vi "X stage safety.vi"(7 "new position":dbl format="%#_13g", 8 "Error In":errorcluster, 10 "Table Stages":T1={"X Stage"={"Position"=0.0, "Is.Enabled?"=FALSE, "Is.Connected?"=FALSE, "Device SN"="45876539", "AccelerationMaximum"=0.0, "VelocityMaximum"=0.0, "Acceleration"=0.0, "Velocity"=0.0, "waitTimeout (ms)"=0, "Model"=enum."None", "Is.Homed?"=FALSE, "MOVE"=FALSE}, "Y Stage"={"Position"=0.0, "Is.Enabled?"=FALSE, "Is.Connected?"=FALSE, "Device SN"="45876539", "AccelerationMaximum"=0.0, "VelocityMaximum"=0.0, "Acceleration"=0.0, "Velocity"=0.0, "waitTimeout (ms)"=0, "Model"=enum."None", "Is.Homed?"=FALSE, "MOVE"=FALSE}, "Z Stage"={"Position"=0.0, "Is.Enabled?"=FALSE, "Is.Connected?"=FALSE, "Device SN"="45876539", "AccelerationMaximum"=0.0, "VelocityMaximum"=0.0, "Acceleration"=0.0, "Velocity"=0.0, "waitTimeout (ms)"=0, "Model"=enum."None", "Is.Homed?"=FALSE, "MOVE"=FALSE}, "Attenuator"={"Position"=0.0, "Is.Enabled?"=FALSE, "Is.Connected?"=FALSE, "Device SN"="45876539", "AccelerationMaximum"=0.0, "VelocityMaximum"=0.0, "Acceleration"=0.0, "Velocity"=0.0, "waitTimeout (ms)"=0, "Model"=enum."None", "Is.Homed?"=FALSE, "MOVE"=FALSE}}) -> (0 "Error Out":errorcluster, 1 "crash?":bool, 2 "Table Stages [out]":T1={"X Stage"={"Position"=0.0, "Is.Enabled?"=FALSE, "Is.Connected?"=FALSE, "Device SN"="45876539", "AccelerationMaximum"=0.0, "VelocityMaximum"=0.0, "Acceleration"=0.0, "Velocity"=0.0, "waitTimeout (ms)"=0, "Model"=enum."None", "Is.Homed?"=FALSE, "MOVE"=FALSE}, "Y Stage"={"Position"=0.0, "Is.Enabled?"=FALSE, "Is.Connected?"=FALSE, "Device SN"="45876539", "AccelerationMaximum"=0.0, "VelocityMaximum"=0.0, "Acceleration"=0.0, "Velocity"=0.0, "waitTimeout (ms)"=0, "Model"=enum."None", "Is.Homed?"=FALSE, "MOVE"=FALSE}, "Z Stage"={"Position"=0.0, "Is.Enabled?"=FALSE, "Is.Connected?"=FALSE, "Device SN"="45876539", "AccelerationMaximum"=0.0, "VelocityMaximum"=0.0, "Acceleration"=0.0, "Velocity"=0.0, "waitTimeout (ms)"=0, "Model"=enum."None", "Is.Homed?"=FALSE, "MOVE"=FALSE}, "Attenuator"={"Position"=0.0, "Is.Enabled?"=FALSE, "Is.Connected?"=FALSE, "Device SN"="45876539", "AccelerationMaximum"=0.0, "VelocityMaximum"=0.0, "Acceleration"=0.0, "Velocity"=0.0, "waitTimeout (ms)"=0, "Model"=enum."None", "Is.Homed?"=FALSE, "MOVE"=FALSE}})   [LabVIEW 2018]
uses:
  Controls/Translation Stage Parameters.ctl
  Hardware Mfg/Thorlabs Translation Stages/Controls/Translation Stage Cluster.ctl
  Controls/Translation Stage Types.ctl
  Controls/Set Get Controls.ctl
  Hardware Mfg/Thorlabs Translation Stages/Controls/Motion Translation Module Control2.ctl
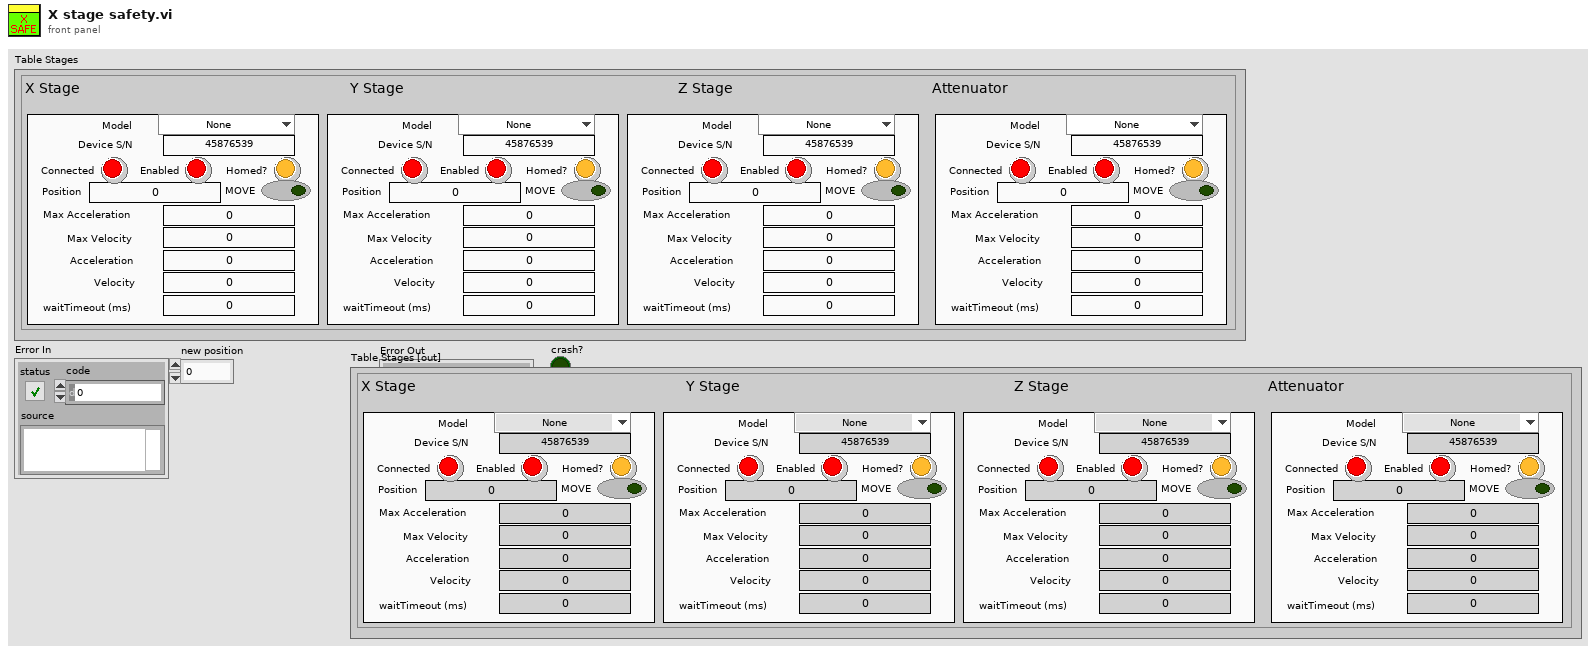
[diagram p1: front panel]
types:
  T1 = typedef "Translation Stage Parameters.ctl" = cluster{"X Stage":T2, "Y Stage":T2, "Z Stage":T2, "Attenuator":T2}
  T2 = typedef "Translation Stage Cluster.ctl" = cluster{"Position":dbl, "Is.Enabled?":bool, "Is.Connected?":bool, "Device SN":string, "AccelerationMaximum":dbl, "VelocityMaximum":dbl, "Acceleration":dbl, "Velocity":dbl, "waitTimeout (ms)":i32, "Model":T3, "Is.Homed?":bool, "MOVE":bool}
  T3 = typedef "Translation Stage Types.ctl" = enum16{"None", "Thorlabs LTS", "Thorlabs MLJ"}
  T4 = typedef "Motion Translation Module Control2.ctl" = enum16{"Init", "Home", "Status", "Velocity/Accel", "Position", "Jog", "Stop", "Uninit", "Enable", "Disable"}
  T5 = typedef "Set Get Controls.ctl" = enum16{"Set", "Get"}
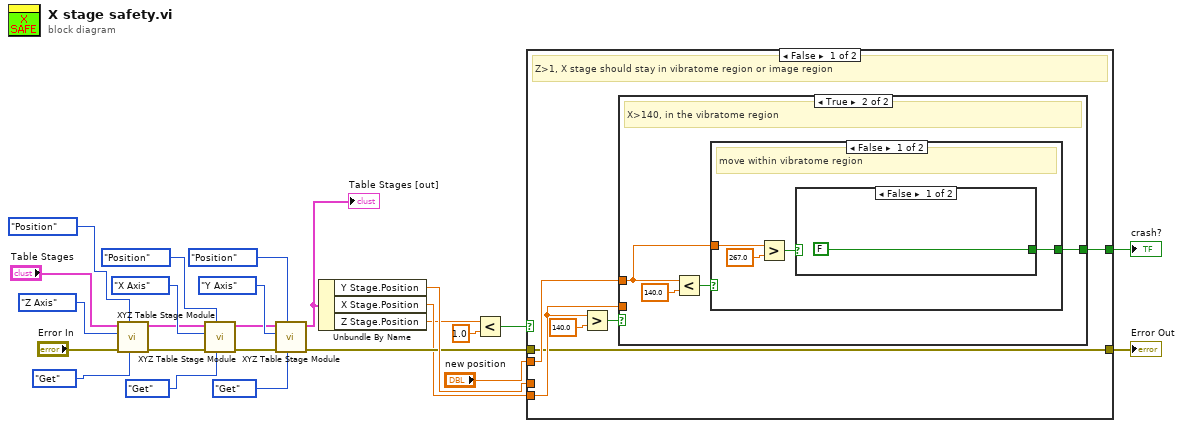
[diagram p0: block diagram]
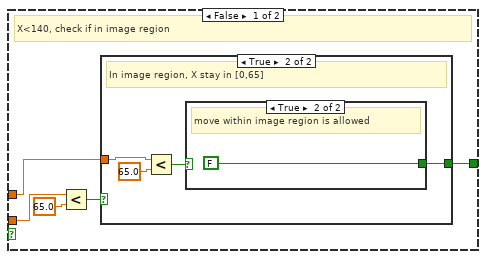
[diagram p2: hidden frame]
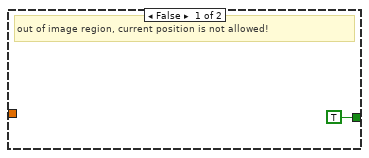
[diagram p3: hidden frame]
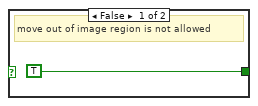
[diagram p4: hidden frame]
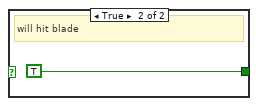
[diagram p5: hidden frame]
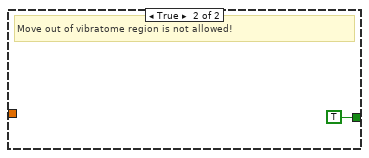
[diagram p6: hidden frame]
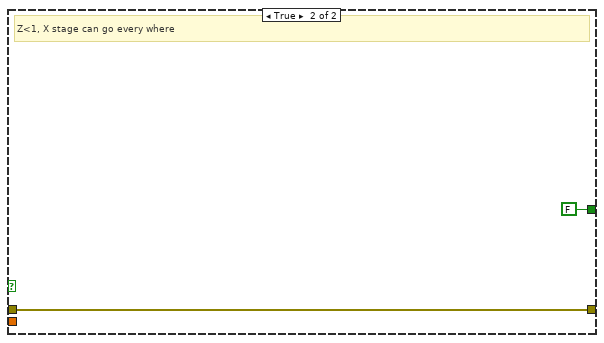
[diagram p7: hidden frame]
diagram:
  n1 = call "XYZ Table Stage Module.vi"("Set/Get"=Set_Get_Controls."Get", "Action"=Motion_Translation_Module_Control2."Position", "Error In"="Error In", "Axis"=enum16{"X Axis", "Y Axis", "Z Axis"}."Z Axis", "Table Stages"="Table Stages") -> ("Error Out"=w18:errorcluster, "Table Stages [out]"=w4:T1)  [unwired: 5 in]
  n2 = call "XYZ Table Stage Module.vi"("Set/Get"=Set_Get_Controls."Get", "Action"=Motion_Translation_Module_Control2."Position", "Error In"=w18, "Axis"=enum16{"X Axis", "Y Axis", "Z Axis"}."X Axis", "Table Stages"=w4) -> ("Error Out"=w14:errorcluster, "Table Stages [out]"=w3:T1)  [unwired: 5 in]
  n3 = call "XYZ Table Stage Module.vi"("Set/Get"=Set_Get_Controls."Get", "Action"=Motion_Translation_Module_Control2."Position", "Error In"=w14, "Axis"=enum16{"X Axis", "Y Axis", "Z Axis"}."Y Axis", "Table Stages"=w3) -> ("Error Out"=w6:errorcluster, "Table Stages [out]"=w13:T1)  [unwired: 5 in]
  "Table Stages [out]" <- w13
  n4 = Unbundle By Name(w13) -> ("Y Stage.Position"=w9:dbl, "X Stage.Position"=w2:dbl, "Z Stage.Position"=w1:dbl)
  n5 = Less?(x=w1, y=1.0) -> (x < y?=w11:bool)
  n6 = case shown="False" w11 {
    tunnel: "new position" -> [w29 _]
    tunnel: w9 -> [_ _]
    tunnel: [w27 FALSE] -> w8
    tunnel: w2 -> [w28 _]
    tunnel: w6 -> [w26 w55]
    tunnel: [w26 w55] -> w5
    frame False {
      # "Z>1, X stage should stay in vibratome region or image region"
      n7 = Greater?(x=w28, y=140.0) -> (0:w30:bool)
      n8 = case shown="True" w30 {
        tunnel: w29 -> [w32 w44]
        tunnel: [w33 w45] -> w27
        tunnel: w28 -> [w36 _]
        frame False {
          # "X<140, check if in image region"
          n9 = Less?(x=w36, y=65.0) -> (x < y?=w34:bool)
          n10 = case shown="True" w34 {
            tunnel: [TRUE w38] -> w33
            tunnel: w32 -> [_ w41]
            frame False {
              # "out of image region, current position is not allowed!"
            }
            frame True {
              # "In image region, X stay in [0,65]"
              n11 = Less?(x=w41, y=65.0) -> (x < y?=w39:bool)
              n12 = case shown="True" w39 {
                tunnel: [TRUE FALSE] -> w38
                frame False {
                  # "move out of image region is not allowed"
                }
                frame True {
                  # "move within image region is allowed"
                }
              }
            }
          }
        }
        frame True {
          # "X>140, in the vibratome region"
          n13 = Less?(x=w44, y=140.0) -> (x < y?=w46:bool)
          n14 = case shown="False" w46 {
            tunnel: [w51 TRUE] -> w45
            tunnel: w44 -> [w50 _]
            frame False {
              # "move within vibratome region"
              n15 = Greater?(x=w50, y=267.0) -> (0:w48:bool)
              n16 = case shown="False" w48 {
                tunnel: [FALSE TRUE] -> w51
                frame False {
                }
                frame True {
                  # "will hit blade"
                }
              }
            }
            frame True {
              # "Move out of vibratome region is not allowed!"
            }
          }
        }
      }
    }
    frame True {
      # "Z<1, X stage can go every where"
    }
  }
  "crash?" <- w8
  "Error Out" <- w5
